vi "校准配置界面.vi"() -> ()   [LabVIEW 2016]
panel:
  out "公式、校准输出":T1={"公式"={"X^2"=0.0, "X"=nan, "B"=nan}, "校准"={"校准？"=FALSE, "校准点1-5"=0, "校准浓度"=0.0}}
  in  "量程下拉列表":enum16{"低量程", "高量程"}(ring)
  in  "确定":bool
  in  "返回":bool
  in  "校准按钮":T2
  in  "曲线模型":T3={"标液浓度1"=0.0, "测量吸光度1"=0.0, "样品1启用"=FALSE, "标液浓度2"=0.0, "测量吸光度2"=0.0, "样品2启用"=FALSE, "标液浓度3"=0.0, "测量吸光度3"=0.0, "样品3启用"=FALSE, "标液浓度4"=0.0, "测量吸光度4"=0.0, "样品4启用"=FALSE, "标液浓度5"=0.0, "测量吸光度5"=0.0, "样品5启用"=FALSE, "模型"=enum."线性", "method"=enum."最小二乘", "精度"=7.0, "XY图"=[], "拟合公式"="", "r^2"=0.0, "零点校准时间"=timestamp(0 s since 1904-01-01), "标液校准时间1"=timestamp(0 s since 1904-01-01), "标液校准时间2"=timestamp(0 s since 1904-01-01), "标液校准时间3"=timestamp(0 s since 1904-01-01), "标液校准时间4"=timestamp(0 s since 1904-01-01)} {"标液校准时间4" format="%<%Y/%m/%d %H:%M:%S>T"; "标液校准时间3" format="%<%Y/%m/%d %H:%M:%S>T"; "标液校准时间2" format="%<%Y/%m/%d %H:%M:%S>T"; "标液校准时间1" format="%<%Y/%m/%d %H:%M:%S>T"; "零点校准时间" format="%<%Y/%m/%d %H:%M:%S>T"; "r^2" format="%.7g"; "标液浓度5" format="%#.2f"; "测量吸光度5" format="%#.0f"; "标液浓度4" format="%#.2f"; "测量吸光度4" format="%#.0f"; "标液浓度3" format="%#.2f"; "测量吸光度3" format="%#.0f"; "标液浓度2" format="%#.2f"; "测量吸光度2" format="%#.0f"; "测量吸光度1" format="%#.0f"; "标液浓度1" format="%#.2f"}
  # "校准模式"
  # "校准时间"
  # "标液浓度"
  # "滴定数显示"
  # "标液1"
  # "标液2"
  # "标液3"
  # "零点"
  # "跨度"
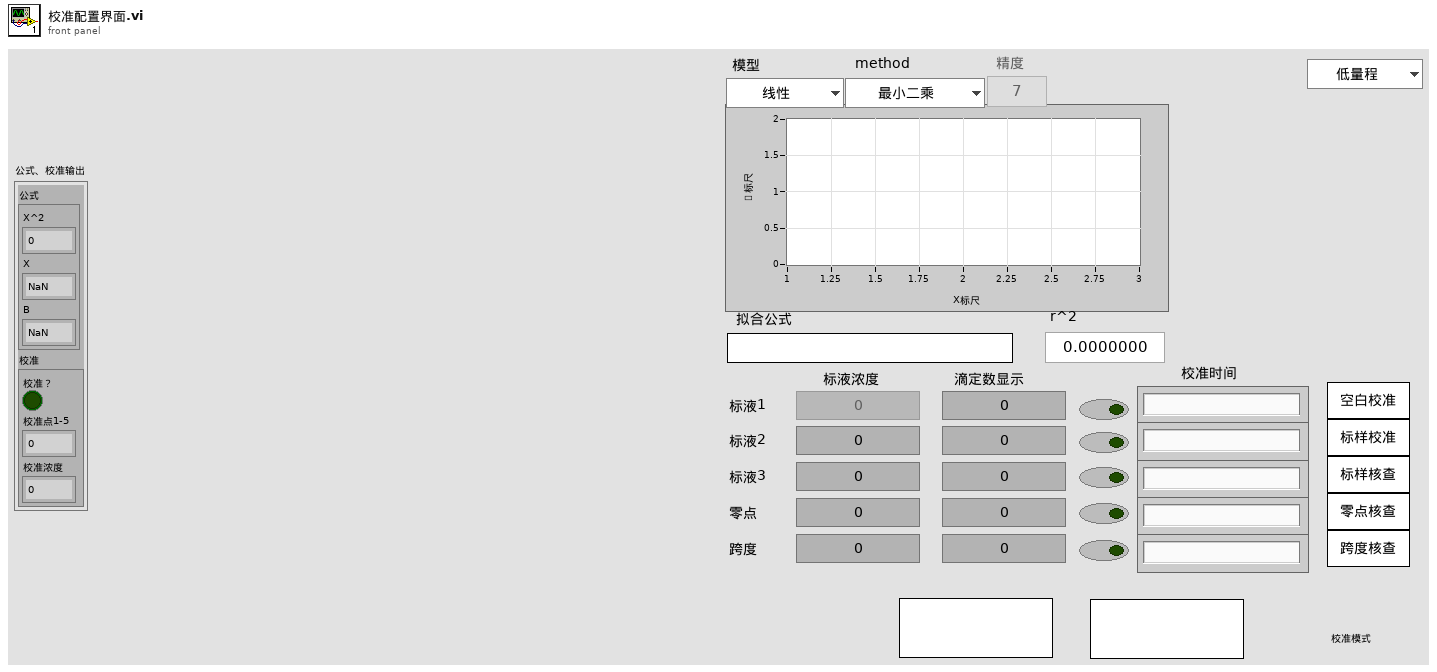
[diagram p1: front panel]
types:
  T1 = cluster{"公式":cluster{"X^2":dbl, "X":dbl, "B":dbl}, "校准":cluster{"校准？":bool, "校准点1-5":u16, "校准浓度":dbl}}
  T2 = cluster{"校准1":bool, "校准2":bool, "校准3":bool, "校准4":bool, "校准5":bool}
  T3 = cluster{"标液浓度1":dbl, "测量吸光度1":dbl, "样品1启用":bool, "标液浓度2":dbl, "测量吸光度2":dbl, "样品2启用":bool, "标液浓度3":dbl, "测量吸光度3":dbl, "样品3启用":bool, "标液浓度4":dbl, "测量吸光度4":dbl, "样品4启用":bool, "标液浓度5":dbl, "测量吸光度5":dbl, "样品5启用":bool, "模型":enum32{"线性", "多项式"}, "method":enum16{"最小二乘", "最小绝对残差", "Bisquare"}, "精度":dbl, "XY图":cluster{"X Values":dbl[], "Y Values":dbl[]}[], "拟合公式":string, "r^2":dbl, "零点校准时间":timestamp, "标液校准时间1":timestamp, "标液校准时间2":timestamp, "标液校准时间3":timestamp, "标液校准时间4":timestamp}
  T4 = enum8{"Enabled", "Disabled", "Disabled and Grayed Out"}
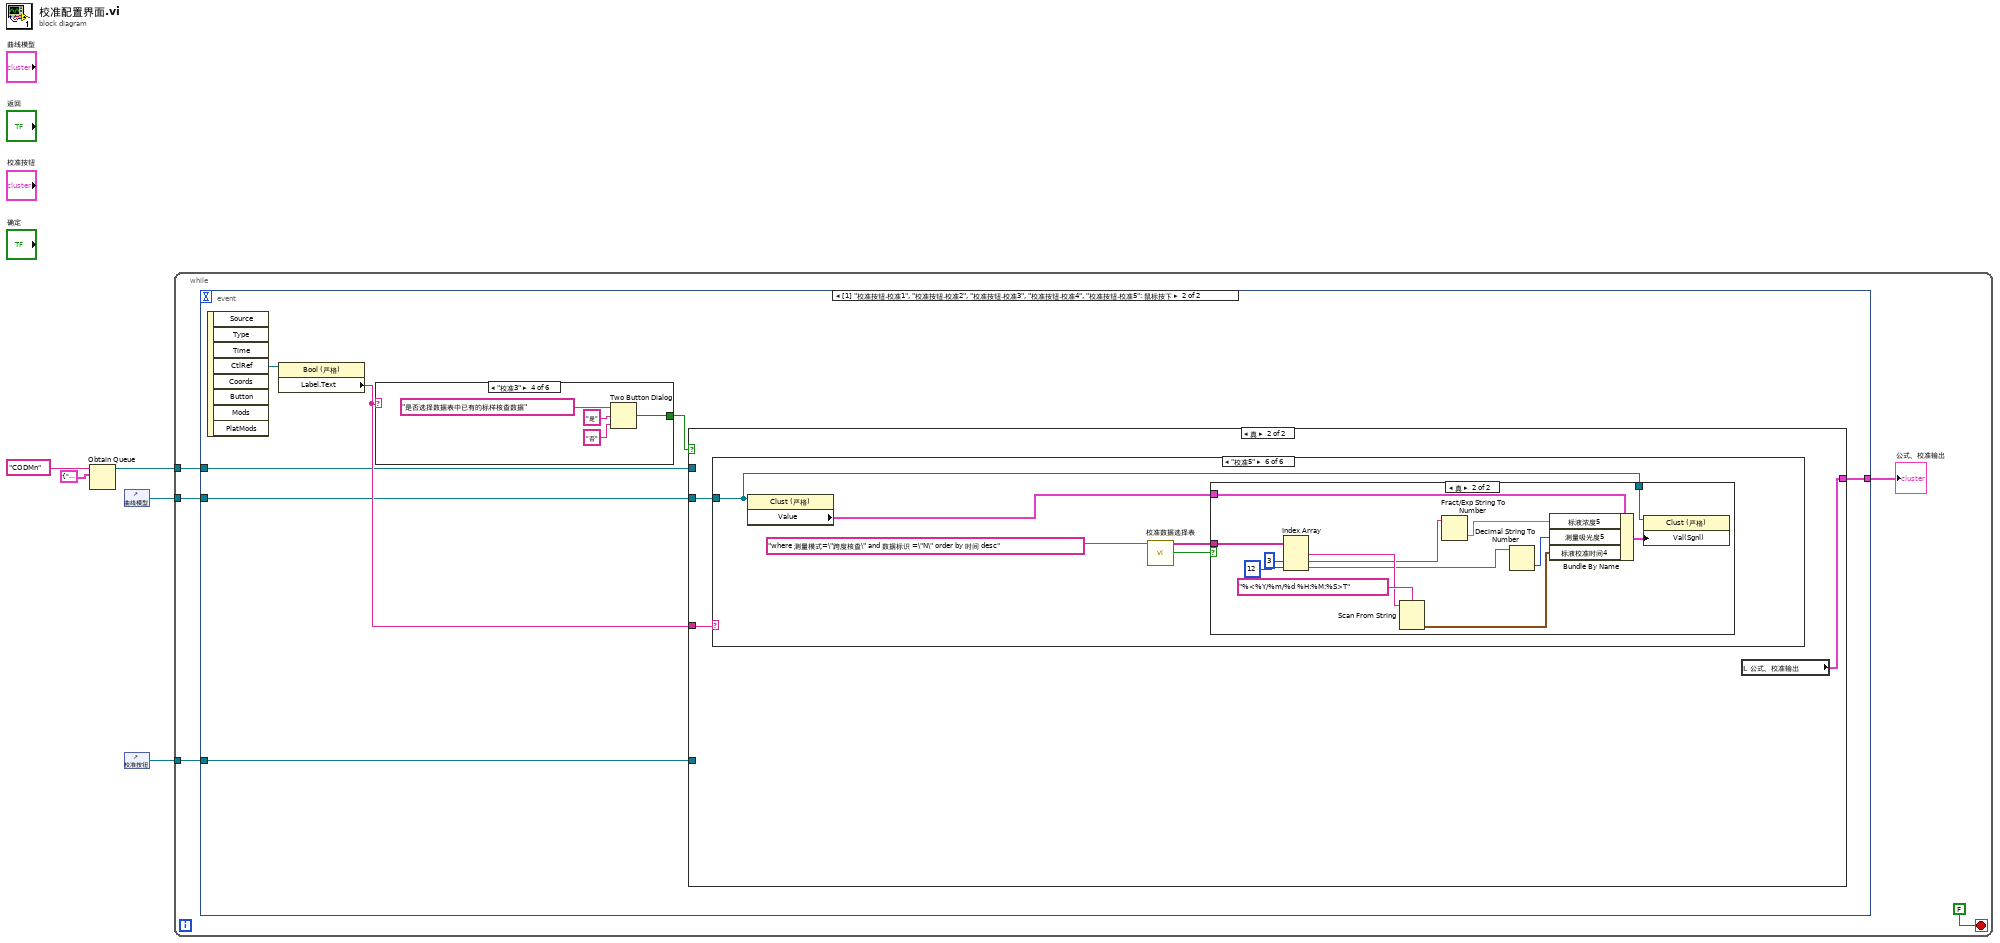
[diagram p0: block diagram]
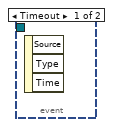
[diagram p2: hidden frame]
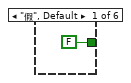
[diagram p3: hidden frame]
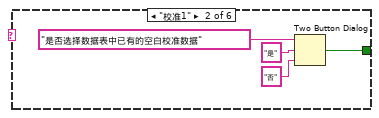
[diagram p4: hidden frame]
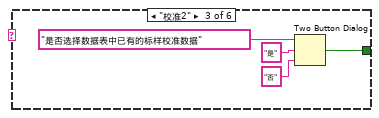
[diagram p5: hidden frame]
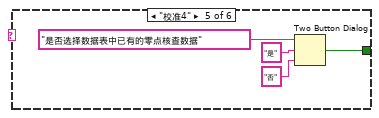
[diagram p6: hidden frame]
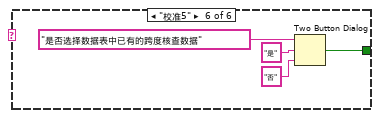
[diagram p7: hidden frame]
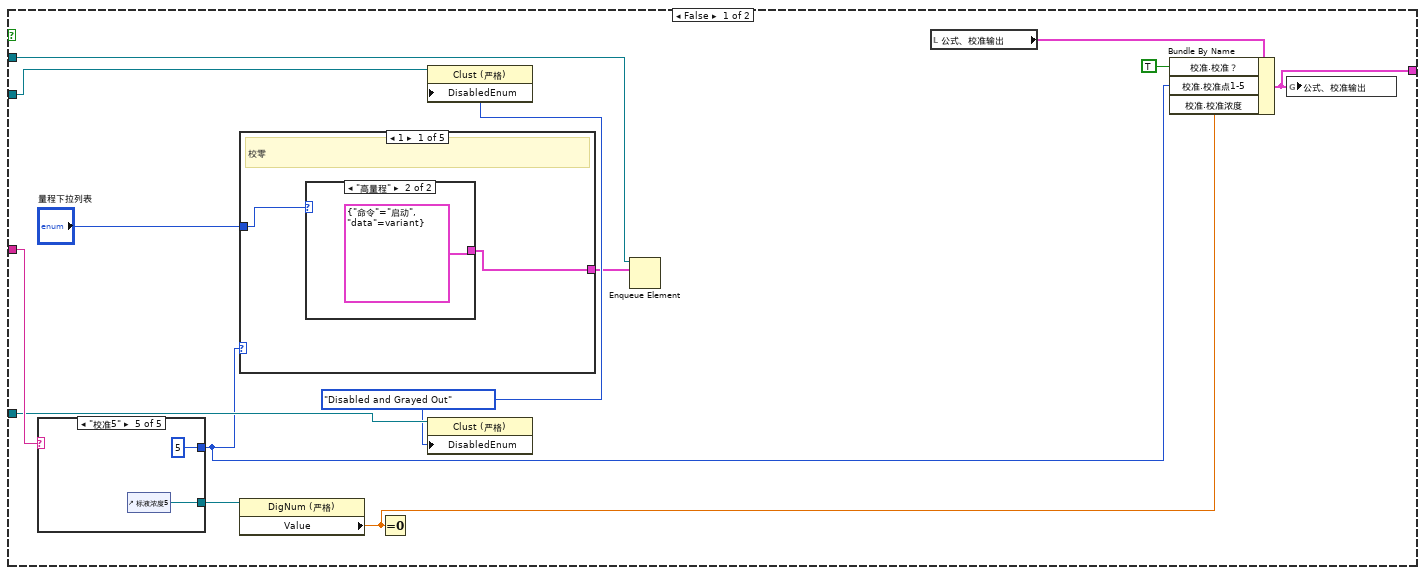
[diagram p8: hidden frame]
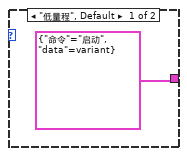
[diagram p9: hidden frame]
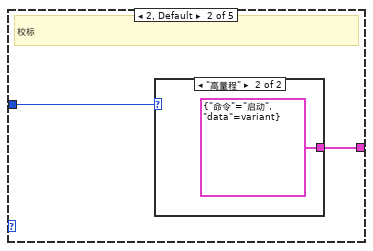
[diagram p10: hidden frame]
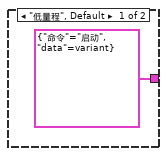
[diagram p11: hidden frame]
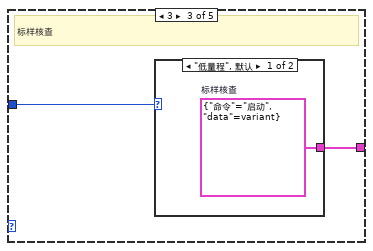
[diagram p12: hidden frame]
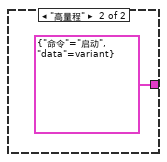
[diagram p13: hidden frame]
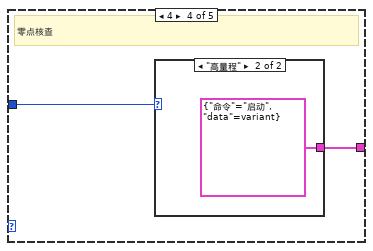
[diagram p14: hidden frame]
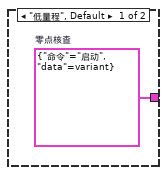
[diagram p15: hidden frame]
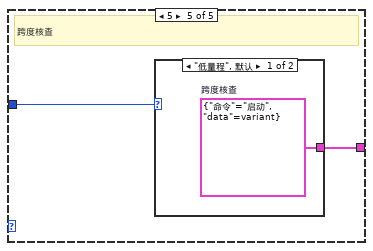
[diagram p16: hidden frame]
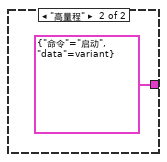
[diagram p17: hidden frame]
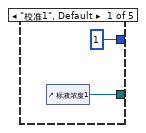
[diagram p18: hidden frame]
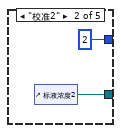
[diagram p19: hidden frame]
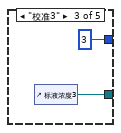
[diagram p20: hidden frame]
diagram:
  n1 = Obtain Queue(name (unnamed)="CODMn" ("名称（未命名）"), element data type=cluster{"命令":string, "data":variant} {"命令"="", "data"=variant}) -> (queue out=w1:refnum<queue>)  [unwired: 3 in, 2 out]
  n2 = control-ref of="曲线模型"() -> (w4:refnum<vi>)
  n3 = control-ref of="校准按钮"() -> (w5:refnum<vi>)
  n4 = while {
    tunnel: w5 -> [w9]
    tunnel: w4 -> [w8]
    tunnel: w1 -> [w7]
    stop <- FALSE stop-if-true
    n5 = event shown="[1] \"校准按钮.校准1\", \"校准按钮.校准2\", \"校准按钮.校准3\", \"校准按钮.校准4\", \"校准按钮.校准5\": 鼠标按下" {
      selector: _ -> [_ _]
      dyn-events: _ -> [_ _]
      timeout: _ -> [_ _]
      tunnel: w9 -> [_ w14]
      tunnel: w8 -> [_ w13]
      tunnel: w7 -> [_ w12]
      tunnel: [_ w11] -> w6
      event Timeout {
        n6 = event-data() -> ()  [unwired: 1 in, 3 out]
      }
      event "校准按钮.校准1", "校准按钮.校准2", "校准按钮.校准3", "校准按钮.校准4", "校准按钮.校准5": Mouse Down {
        n7 = event-data() -> ("CtlRef"=w15:refnum<vi>)  [unwired: 1 in, 7 out]
        n8 = property class="Bool (严格)"(reference=w15) -> ("Label.Text"=w16:string)  [unwired: 1 in, 2 out]
        n9 = case shown="\"校准3\"" w16 {
          tunnel: [FALSE ("T button?") w19 w23 w27 w31 w35] -> w17
          frame "假", Default {
          }
          frame "校准1" {
            n10 = Two Button Dialog(message="是否选择数据表中已有的空白校准数据" ("消息"), 1:"否" ("F按钮名称（“取消”）"), 2:"是" ("T按钮名称（“确定”）")) -> (T button?=w19:bool)
          }
          frame "校准2" {
            n11 = Two Button Dialog(message="是否选择数据表中已有的标样校准数据" ("消息"), 1:"否" ("F按钮名称（“取消”）"), 2:"是" ("T按钮名称（“确定”）")) -> (T button?=w23:bool)
          }
          frame "校准3" {
            n12 = Two Button Dialog(message="是否选择数据表中已有的标样核查数据" ("消息"), 1:"否" ("F按钮名称（“取消”）"), 2:"是" ("T按钮名称（“确定”）")) -> (T button?=w27:bool)
          }
          frame "校准4" {
            n13 = Two Button Dialog(message="是否选择数据表中已有的零点核查数据" ("消息"), 1:"否" ("F按钮名称（“取消”）"), 2:"是" ("T按钮名称（“确定”）")) -> (T button?=w31:bool)
          }
          frame "校准5" {
            n14 = Two Button Dialog(message="是否选择数据表中已有的跨度核查数据" ("消息"), 1:"否" ("F按钮名称（“取消”）"), 2:"是" ("T按钮名称（“确定”）")) -> (T button?=w35:bool)
          }
        }
        n15 = case shown="真" w17 {
          tunnel: w16 -> [w51 w83]
          tunnel: w13 -> [w47 w84]
          tunnel: w14 -> [w46 _]
          tunnel: w12 -> [w42 _]
          tunnel: [w41 w82] -> w11
          frame False {
            w45 = T4."Disabled and Grayed Out" ("禁用")
            n16 = case shown="\"校准5\"" w51 {
              tunnel: [w72 w74 w76 w78 w80] -> w49
              tunnel: [u16 1 ("校准点1-5") u16 2 ("校准点1-5") u16 3 ("校准点1-5") u16 4 ("校准点1-5") u16 5 ("校准点1-5")] -> w40
              frame "校准1", Default {
                n17 = control-ref of="标液浓度1"() -> (w72:refnum<vi>)
              }
              frame "校准2" {
                n18 = control-ref of="标液浓度2"() -> (w74:refnum<vi>)
              }
              frame "校准3" {
                n19 = control-ref of="标液浓度3"() -> (w76:refnum<vi>)
              }
              frame "校准4" {
                n20 = control-ref of="标液浓度4"() -> (w78:refnum<vi>)
              }
              frame "校准5" {
                n21 = control-ref of="标液浓度5"() -> (w80:refnum<vi>)
              }
            }
            n22 = case shown="1" w40 {
              tunnel: [w53 w56 w60 w64 w68] -> w43
              tunnel: "量程下拉列表" -> [w52 w57 w61 w65 w69]
              frame 1 {
                # "校零"
                n23 = case shown="\"高量程\"" w52 {
                  tunnel: [cluster{"命令":string, "data":variant} {"命令"="启动", "data"=variant(cluster{"站号":u16, "控制命令":u16[]} {"站号"=21, "控制命令"=[2048, 0]})} ("元素") cluster{"命令":string, "data":variant} {"命令"="启动", "data"=variant(cluster{"站号":u16, "控制命令":u16[]} {"站号"=21, "控制命令"=[2048, 256]})} ("元素")] -> w53
                  frame "低量程", Default {
                  }
                  frame "高量程" {
                  }
                }
              }
              frame 2, Default {
                # "校标"
                n24 = case shown="\"高量程\"" w57 {
                  tunnel: [cluster{"命令":string, "data":variant} {"命令"="启动", "data"=variant(cluster{"站号":u16, "控制命令":u16[]} {"站号"=21, "控制命令"=[2304, 0]})} ("元素") cluster{"命令":string, "data":variant} {"命令"="启动", "data"=variant(cluster{"站号":u16, "控制命令":u16[]} {"站号"=21, "控制命令"=[2304, 256]})} ("元素")] -> w56
                  frame "低量程", Default {
                  }
                  frame "高量程" {
                  }
                }
              }
              frame 3 {
                # "标样核查"
                n25 = case shown="\"低量程\", 默认" w61 {
                  tunnel: [w62 cluster{"命令":string, "data":variant} {"命令"="启动", "data"=variant(cluster{"站号":u16, "控制命令":u16[]} {"站号"=21, "控制命令"=[512, 256]})} ("元素")] -> w60
                  frame "低量程", Default {
                    w62 = cluster{"命令":string, "data":variant} {"命令"="启动", "data"=variant(cluster{"站号":u16, "控制命令":u16[]} {"站号"=21, "控制命令"=[512, 0]})}  # 标样核查
                  }
                  frame "高量程" {
                  }
                }
              }
              frame 4 {
                # "零点核查"
                n26 = case shown="\"高量程\"" w65 {
                  tunnel: [w66 cluster{"命令":string, "data":variant} {"命令"="启动", "data"=variant(cluster{"站号":u16, "控制命令":u16[]} {"站号"=21, "控制命令"=[768, 256]})} ("元素")] -> w64
                  frame "低量程", Default {
                    w66 = cluster{"命令":string, "data":variant} {"命令"="启动", "data"=variant(cluster{"站号":u16, "控制命令":u16[]} {"站号"=21, "控制命令"=[768, 0]})}  # 零点核查
                  }
                  frame "高量程" {
                  }
                }
              }
              frame 5 {
                # "跨度核查"
                n27 = case shown="\"低量程\", 默认" w69 {
                  tunnel: [w70 cluster{"命令":string, "data":variant} {"命令"="启动", "data"=variant(cluster{"站号":u16, "控制命令":u16[]} {"站号"=21, "控制命令"=[1024, 256]})} ("元素")] -> w68
                  frame "低量程", Default {
                    w70 = cluster{"命令":string, "data":variant} {"命令"="启动", "data"=variant(cluster{"站号":u16, "控制命令":u16[]} {"站号"=21, "控制命令"=[1024, 0]})}  # 跨度核查
                  }
                  frame "高量程" {
                  }
                }
              }
            }
            n28 = property class="DigNum (严格)"(reference=w49) -> ("Value"=w44:dbl)  [unwired: 1 in, 2 out]
            n29 = Equal To 0?(x=w44) -> ()  [unwired: 1 out]
            n30 = property class="Clust (严格)"(reference=w47, "DisabledEnum"=w45) -> ()  [unwired: 1 in, 2 out]
            n31 = property class="Clust (严格)"(reference=w46, "DisabledEnum"=w45) -> ()  [unwired: 1 in, 2 out]
            n32 = Enqueue Element(queue=w42, element=w43) -> ()  [unwired: 2 in, 3 out]
            n33 = local read "公式、校准输出"() -> (w48:T1)
            n34 = Bundle By Name(cluster=w48, "校准.校准？"=TRUE ("校准？"), "校准.校准点1-5"=w40, "校准.校准浓度"=w44) -> (w41:T1)
            n35 = global write "CODMn断电保存全局变量.vi" "公式、校准输出"(w41) -> ()
          }
          frame True {
            n36 = case shown="\"校准5\"" w83 {
              tunnel: w84 -> [_ w89 w107 w125 w143 w161]
              frame "假", Default {
              }
              frame "校准1" {
                n37 = property class="Clust (严格)"(reference=w89) -> ("Value"=w88:T3)  [unwired: 1 in, 2 out]
                n38 = call "校准数据选择表.vi"("condition"="where 测量模式=\"空白校准\" and 数据标识 =\"N\" order by 时间 desc") -> ("布尔"=w85:bool, "ItemNames"=w87:string[])  [unwired: 9 in]
                n39 = case shown="真" w85 {
                  tunnel: w89 -> [_ w102]
                  tunnel: w88 -> [_ w101]
                  tunnel: w87 -> [_ w96]
                  frame False {
                  }
                  frame True {
                    n40 = Index Array(array=w96, index #2=3 ("索引"), index #3=12 ("索引")) -> (element #1=w93:string, element #2=w91:string, element #3=w92:string)  [unwired: 1 in]
                    n41 = Scan From String(format string="%<%Y/%m/%d %H:%M:%S>T" ("格式字符串"), input string=w93) -> (output 1=w98:timestamp)  [unwired: 3 in, 3 out]
                    n42 = Fract/Exp String To Number(string=w91) -> (number=w90:dbl)  [unwired: 3 in, 1 out]
                    n43 = Decimal String To Number(string=w92) -> (number=w97:i32)  [unwired: 2 in, 1 out]
                    n44 = Bundle By Name(cluster=w101, "标液浓度1"=w90, "测量吸光度1"=w97, "零点校准时间"=w98) -> (w100:T3)
                    n45 = property class="Clust (严格)"(reference=w102, "Val(Sgnl)"=w100) -> ()  [unwired: 1 in, 2 out]
                  }
                }
              }
              frame "校准2" {
                n46 = property class="Clust (严格)"(reference=w107) -> ("Value"=w106:T3)  [unwired: 1 in, 2 out]
                n47 = call "校准数据选择表.vi"("condition"="where 测量模式=\"标样校准\" and 数据标识 =\"N\" order by 时间 desc") -> ("布尔"=w103:bool, "ItemNames"=w105:string[])  [unwired: 9 in]
                n48 = case shown="真" w103 {
                  tunnel: w107 -> [_ w120]
                  tunnel: w106 -> [_ w119]
                  tunnel: w105 -> [_ w114]
                  frame False {
                  }
                  frame True {
                    n49 = Index Array(array=w114, index #2=3 ("索引"), index #3=12 ("索引")) -> (element #1=w111:string, element #2=w109:string, element #3=w110:string)  [unwired: 1 in]
                    n50 = Scan From String(format string="%<%Y/%m/%d %H:%M:%S>T" ("格式字符串"), input string=w111) -> (output 1=w116:timestamp)  [unwired: 3 in, 3 out]
                    n51 = Fract/Exp String To Number(string=w109) -> (number=w108:dbl)  [unwired: 3 in, 1 out]
                    n52 = Decimal String To Number(string=w110) -> (number=w115:i32)  [unwired: 2 in, 1 out]
                    n53 = Bundle By Name(cluster=w119, "标液浓度2"=w108, "测量吸光度2"=w115, "标液校准时间1"=w116) -> (w118:T3)
                    n54 = property class="Clust (严格)"(reference=w120, "Val(Sgnl)"=w118) -> ()  [unwired: 1 in, 2 out]
                  }
                }
              }
              frame "校准3" {
                n55 = property class="Clust (严格)"(reference=w125) -> ("Value"=w124:T3)  [unwired: 1 in, 2 out]
                n56 = call "校准数据选择表.vi"("condition"="where 测量模式=\"标样核查\" and 数据标识 =\"N\" order by 时间 desc") -> ("布尔"=w121:bool, "ItemNames"=w122:string[])  [unwired: 9 in]
                n57 = case shown="真" w121 {
                  tunnel: w125 -> [_ w138]
                  tunnel: w124 -> [_ w137]
                  tunnel: w122 -> [_ w129]
                  frame False {
                  }
                  frame True {
                    n58 = Index Array(array=w129, index #2=3 ("索引"), index #3=12 ("索引")) -> (element #1=w128:string, element #2=w127:string, element #3=w126:string)  [unwired: 1 in]
                    n59 = Scan From String(format string="%<%Y/%m/%d %H:%M:%S>T" ("格式字符串"), input string=w128) -> (output 1=w134:timestamp)  [unwired: 3 in, 3 out]
                    n60 = Fract/Exp String To Number(string=w127) -> (number=w133:dbl)  [unwired: 3 in, 1 out]
                    n61 = Decimal String To Number(string=w126) -> (number=w132:i32)  [unwired: 2 in, 1 out]
                    n62 = Bundle By Name(cluster=w137, "标液浓度3"=w133, "测量吸光度3"=w132, "标液校准时间2"=w134) -> (w136:T3)
                    n63 = property class="Clust (严格)"(reference=w138, "Val(Sgnl)"=w136) -> ()  [unwired: 1 in, 2 out]
                  }
                }
              }
              frame "校准4" {
                n64 = property class="Clust (严格)"(reference=w143) -> ("Value"=w142:T3)  [unwired: 1 in, 2 out]
                n65 = call "校准数据选择表.vi"("condition"="where 测量模式=\"零点核查\" and 数据标识 =\"N\" order by 时间 desc") -> ("布尔"=w139:bool, "ItemNames"=w140:string[])  [unwired: 9 in]
                n66 = case shown="真" w139 {
                  tunnel: w143 -> [_ w156]
                  tunnel: w142 -> [_ w155]
                  tunnel: w140 -> [_ w148]
                  frame False {
                  }
                  frame True {
                    n67 = Index Array(array=w148, index #2=3 ("索引"), index #3=12 ("索引")) -> (element #1=w147:string, element #2=w145:string, element #3=w146:string)  [unwired: 1 in]
                    n68 = Scan From String(format string="%<%Y/%m/%d %H:%M:%S>T" ("格式字符串"), input string=w147) -> (output 1=w152:timestamp)  [unwired: 3 in, 3 out]
                    n69 = Fract/Exp String To Number(string=w145) -> (number=w144:dbl)  [unwired: 3 in, 1 out]
                    n70 = Decimal String To Number(string=w146) -> (number=w151:i32)  [unwired: 2 in, 1 out]
                    n71 = Bundle By Name(cluster=w155, "标液浓度4"=w144, "测量吸光度4"=w151, "标液校准时间3"=w152) -> (w154:T3)
                    n72 = property class="Clust (严格)"(reference=w156, "Val(Sgnl)"=w154) -> ()  [unwired: 1 in, 2 out]
                  }
                }
              }
              frame "校准5" {
                n73 = property class="Clust (严格)"(reference=w161) -> ("Value"=w160:T3)  [unwired: 1 in, 2 out]
                n74 = call "校准数据选择表.vi"("condition"="where 测量模式=\"跨度核查\" and 数据标识 =\"N\" order by 时间 desc") -> ("布尔"=w157:bool, "ItemNames"=w158:string[])  [unwired: 9 in]
                n75 = case shown="真" w157 {
                  tunnel: w161 -> [_ w174]
                  tunnel: w160 -> [_ w173]
                  tunnel: w158 -> [_ w168]
                  frame False {
                  }
                  frame True {
                    n76 = Index Array(array=w168, index #2=3 ("索引"), index #3=12 ("索引")) -> (element #1=w167:string, element #2=w163:string, element #3=w164:string)  [unwired: 1 in]
                    n77 = Scan From String(format string="%<%Y/%m/%d %H:%M:%S>T" ("格式字符串"), input string=w167) -> (output 1=w170:timestamp)  [unwired: 3 in, 3 out]
                    n78 = Fract/Exp String To Number(string=w163) -> (number=w162:dbl)  [unwired: 3 in, 1 out]
                    n79 = Decimal String To Number(string=w164) -> (number=w169:i32)  [unwired: 2 in, 1 out]
                    n80 = Bundle By Name(cluster=w173, "标液浓度5"=w162, "测量吸光度5"=w169, "标液校准时间4"=w170) -> (w172:T3)
                    n81 = property class="Clust (严格)"(reference=w174, "Val(Sgnl)"=w172) -> ()  [unwired: 1 in, 2 out]
                  }
                }
              }
            }
            n82 = local read "公式、校准输出"() -> (w82:T1)
          }
        }
      }
    }
    "公式、校准输出" <- w6
  }
